vi "split_num_uint16_t.vi"(10 "read_frame":string, 11 "id (2 characters)":string) -> (3 "num_uint16_t":u16)   [LabVIEW 2020]
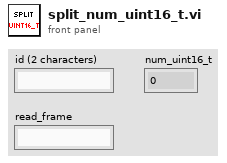
[diagram p1: front panel]
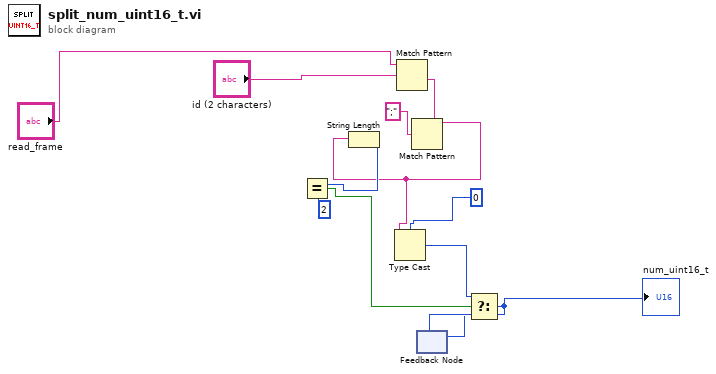
[diagram p0: block diagram]
diagram:
  n1 = Match Pattern(string="read_frame", regular expression="id (2 characters)") -> (after substring=w1:string)  [unwired: 1 in, 3 out]
  n2 = Match Pattern(string=w1, regular expression=";") -> (before substring=w7:string)  [unwired: 1 in, 3 out]
  n3 = String Length(string=w7) -> (length=w8:i32)
  n4 = Equal?(x=w8, y=2) -> (x = y?=w10:bool)
  n5 = Type Cast(type=u16 0, x=w7) -> (*(type *) &x=w4:u16)
  n6 = feedback #1() -> (w5:u16)  [unwired: 1 in]
  n7 = Select(t=w4, s=w10, f=w5) -> (s? t:f=w11:u16)
  "num_uint16_t" <- w11
  n8 = feedback-in #1(w11) -> ()
